vi "Error Bad State.vi"(8 "error in (no error)":errorcluster, 10 "Message":string) -> (0 "error out":errorcluster)   [LabVIEW 2020, in "Stream.lvlib"]
uses:
  Stream.lvlib
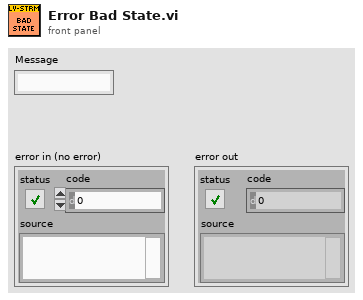
[diagram p1: front panel]
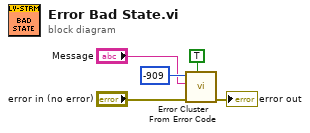
[diagram p0: block diagram]
diagram:
  n1 = call <vilib>:"Error Cluster From Error Code.vi"("show call chain? (False)"=TRUE, "error in (no error)"="error in (no error)", "error message (\"\")"="Message", "error code (0)"=-909) -> ("error out"=→"error out":errorcluster)  [unwired: 5 in]
